vi "JsonFile Load.vi"(8 "error in (no error)":errorcluster, 11 "Path":path) -> (0 "error out":errorcluster, 3 "text":string)   [LabVIEW 2019, in "lv-apt-json-file.lvlib"]
uses:
  lv-apt-json-file.lvlib
  <userlib>/NEVSTOP-Programming-Palette/Configuration/Ini/ini_configuration.lvlib
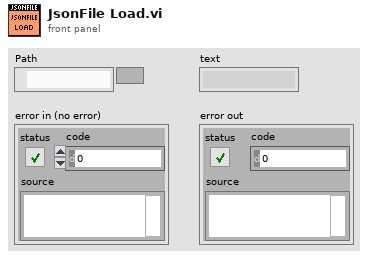
[diagram p1: front panel]
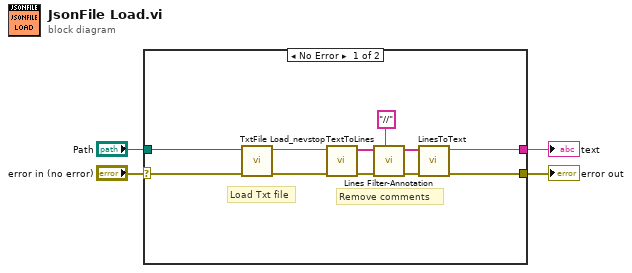
[diagram p0: block diagram]
diagram:
  n1 = case shown="No Error" "error in (no error)" {
    selector: "error in (no error)" -> [w15 w16]
    tunnel: "Path" -> [w14 _]
    tunnel: [w6 _] -> w2
    tunnel: [w5 w16] -> w1
    frame No Error {
      # "Load Txt file"
      # "Remove comments"
      n2 = call <userlib>:"TxtFile Load_nevstop.vi"("error in (no error)"=w15, "Path"=w14) -> ("error out"=w8:errorcluster, "text"=w7:string)  [unwired: 8 in]
      n3 = call <userlib>:"TextToLines.vi"("error in (no error)"=w8, "string"=w7) -> ("error out"=w11:errorcluster, "Lines"=w12:string[])  [unwired: 8 in]
      n4 = call <userlib>:"Lines Filter-Annotation.vi"("Annotation Seperator(#)"="//", "error in (no error)"=w11, "Lines"=w12) -> ("error out"=w9:errorcluster, "Config Text List"=w10:string[])  [unwired: 7 in]
      n5 = call <userlib>:"LinesToText.vi"("error in (no error)"=w9, "Lines"=w10) -> ("error out"=w5:errorcluster, "string"=w6:string)  [unwired: 8 in]
    }
    frame Error {
    }
  }
  "error out" <- w1
  "text" <- w2
